vi "Configure Reference.vi"(0 "VISA resource name":refnum<visa-resource-name>, 1 "Auto Phase (T: Enabled)":bool=TRUE, 2 "Manual Phase (0 Degree)":dbl, 5 "Reference Source (1: Internal)":u16(ring)=1 items=["External", "Internal"], 7 "Sine Output Amplitude (1 V)":dbl=1.0, 9 "Detection Harmonic Number (1)":dbl=1.0, 11 "error in (no error)":errorcluster, 12 "Internal Reference Frequency (1000 Hz)":dbl=1000.0, 13 "External Reference Trigger (0: Sine Zero Crossing)":u16(ring) items=["Sine Zero Crossing", "TTL Rising Edge", "TTL Falling Edge"]) -> (4 "VISA resource name out":refnum<visa-resource-name>, 15 "error out":errorcluster)   [LabVIEW 2020, in "SR830.lvlib"]
doc: "Configures the reference source and the internal oscillator."
uses:
  SR830.lvlib
panel:
  # "Signal Generator"
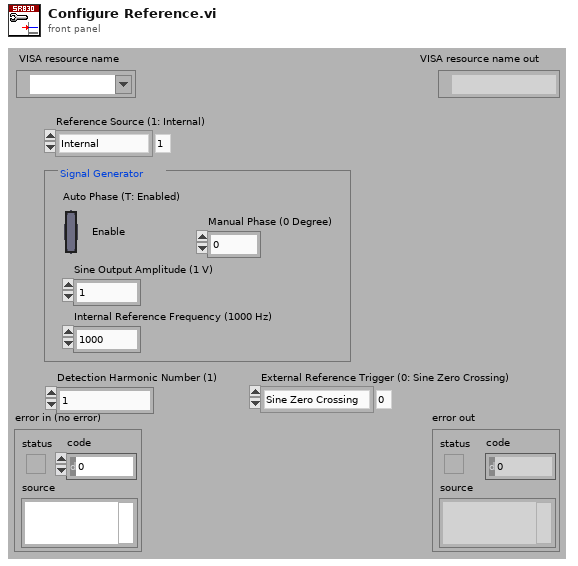
[diagram p1: front panel]
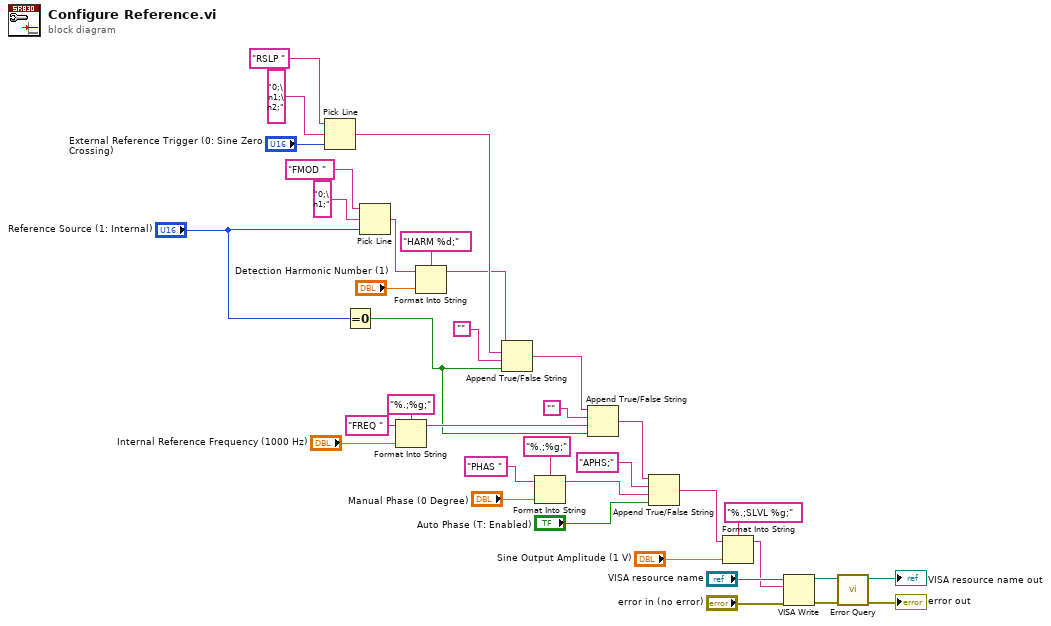
[diagram p0: block diagram]
diagram:
  n1 = Pick Line(string ("")="RSLP ", multi-line string="0;\n1;\n2;", line index="External Reference Trigger (0: Sine Zero Crossing)") -> (output string=w25:string)
  n2 = Equal To 0?(x="Reference Source (1: Internal)") -> (x = 0?=w1:bool)
  n3 = Pick Line(string ("")="FMOD ", multi-line string="0;\n1;", line index="Reference Source (1: Internal)") -> (output string=w31:string)
  n4 = Format Into String(format string="%.;%g;", initial string="FREQ ", "Internal Reference Frequency (1000 Hz)") -> (resulting string=w3:string)  [unwired: 1 in, 1 out]
  n5 = Format Into String(format string="HARM %d;", initial string=w31, "Detection Harmonic Number (1)") -> (resulting string=w23:string)  [unwired: 1 in, 1 out]
  n6 = Append True/False String(1:w1, 2:"" ("false string"), 3:w25, 4:w23) -> (0:w13:string)
  n7 = Format Into String(format string="%.;%g;", initial string="PHAS ", "Manual Phase (0 Degree)") -> (resulting string=w17:string)  [unwired: 1 in, 1 out]
  n8 = Append True/False String(1:w1, 2:w3, 3:"" ("false string"), 4:w13) -> (0:w12:string)
  n9 = Append True/False String(1:"Auto Phase (T: Enabled)", 2:w17, 3:"APHS;" ("true string"), 4:w12) -> (0:w10:string)
  n10 = Format Into String(format string="%.;SLVL %g;", initial string=w10, "Sine Output Amplitude (1 V)") -> (resulting string=w8:string)  [unwired: 1 in, 1 out]
  n11 = VISA Write(VISA resource name="VISA resource name", write buffer=w8, error in (no error)="error in (no error)") -> (VISA resource name out=w7:refnum<visa-resource-name>, error out=w6:errorcluster)  [unwired: 1 out]
  n12 = call "Error Query.vi"("error in (no error)"=w6, "VISA resource name"=w7) -> ("error out"=→"error out":errorcluster, "VISA resource name out"=→"VISA resource name out":refnum<visa-resource-name>)  [unwired: 7 in, 1 out]
